vi "Demo-ReadFile&CRC.vi"() -> ()   [LabVIEW 2016]
panel:
  out "CRC":u32 format="%08x"
  out "error out":errorcluster caption="错误输出"
  in  "Path In":path
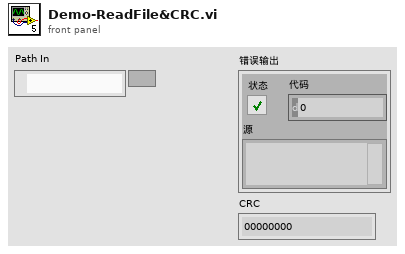
[diagram p1: front panel]
types:
  T1 = typedef "JLINKARM AllDataType.ctl" = cluster{"Addr":u32, "Data":u8[]}
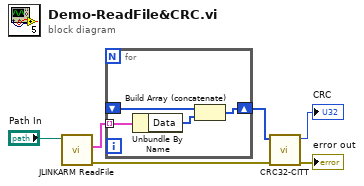
[diagram p0: block diagram]
diagram:
  n1 = call <userlib>:"JLINKARM ReadFile.vi"("Path In"="Path In") -> ("error out"=w6:errorcluster, "Data"=w3:T1[])  [unwired: 6 in, 3 out]
  n2 = for {
    tunnel: w3 -> [w10] mode=indexing
    shift-right: [w7] -> w2
    shift-left: _ -> [w9]
    n3 = Unbundle By Name(w10) -> ("Data"=w8:u8[])
    n4 = Build Array (concatenate)(w9, w8) -> (w7:u8[])
  }
  n5 = call <userlib>:"CRC32-CITT.vi"("error in (no error)"=w6, "Data"=w2) -> ("error out"=→"error out":errorcluster, "CRC"=→"CRC":u32)  [unwired: 8 in]
